vi "MainPanel.vi"() -> ()   [LabVIEW 2015]
uses:
  C:/Users/hskinner-bahay/Documents/GitHub/Kent_State_Project/Labview/LaserControl/SlugHFVInterface/SlugHFVInterface/bin/Debug/SlugHFVInterface.dll
  SlugHFVInterface/SlugHFVInterface/bin/Debug/SlugHFVInterface.dll
  <vilib>/Instr/_visa.llb/VISA Configure Serial Port (Instr).vi
panel:
  in  "Pulse Spacing":u8(knob) max=60 step=10 scale=0.0..60.0
  in  "Pulse Duration":u8(knob) max=60 step=10 scale=0.0..60.0
  in  "Duty Cycle":u8(knob)=100 max=100 step=50 scale=0.0..100.0
  in  "Power Level":u8(knob)=5 max=10 step=1 scale=0.0..10.0
  out "Power On Indicator":u32(colorbox)
  out "Fault LED":bool
  in  "Stop Button 3":bool
  in  "Start Button":bool
  in  "Stop Button":bool
  in  "Load Settings Button":bool
  in  "Saved Settings Field":string(combo)
  in  "Save Settings Button":bool
  in  "Save Settings Field":string
  out "Duty Cycle Slide":u8(slide) scale=0.0..100.0
  out "Slide 2":u8(slide) scale=0.0..100.0
  in  "Load Treatment Field":string(combo)
  in  "Instructions Dialog":bool
  out "Power Level Slide":u8(slide) max=100 step=5 scale=0.0..100.0
  in  "Tab Control":T1(tab)
  out "Strength Slide":u8(slide) scale=0.0..100.0
  out "Internlock LED":bool
  out "Temperature Slide":u8(slide) scale=0.0..100.0
  out "Power On LED":bool
  out "Cooling System LED":bool
  out "RF Active LED":bool
  in  "Numeric":dbl
  in  "Numeric 2":dbl
  in  "OK Button 7":bool
  in  "OK Button 8":bool
  in  "Numeric 3":dbl
  in  "Numeric 4":dbl
  out "Numeric 5":dbl
  out "Numeric 6":dbl
  out "Numeric 7":dbl
  out "Numeric 8":dbl
  in  "String 2":string
  in  "OK Button 5":bool
  in  "HFV Interface":refnum<visa-resource-name>
  # "HFV and Laser Control Panel"
  # "Pulse Duration"
  # "Power On"
  # "Stop"
  # "Power Level"
  # "Duty Cycle"
  # "Pulse Spacing"
  # "Begin Treatment"
  # "Load Treatment"
  # "Settings"
  # "Subject Temperature"
  # "Power On"
  # "Abort"
  # "Warning"
  # "Strength"
  # "Cooling System"
  # "Interlock"
  # "RF Active"
  # "Subject Temperature"
  # "Abort Cutoff (K)"
  # "Warning Cutoff (K)"
  # "Thermo Camera"
  # "Bounding Box"
  # "Measurement Filter (K)"
  # "High"
  # "Low"
  # "Thermo Camera"
  # "Save Readings"
  # "1"
  # "Probes"
  # "2"
  # "3"
  # "HFV Port (COM)"
  # "HFV Interface Circuit (COM)"
  # "Thermo Camera"
  # "Water Chiller Status (COM)"
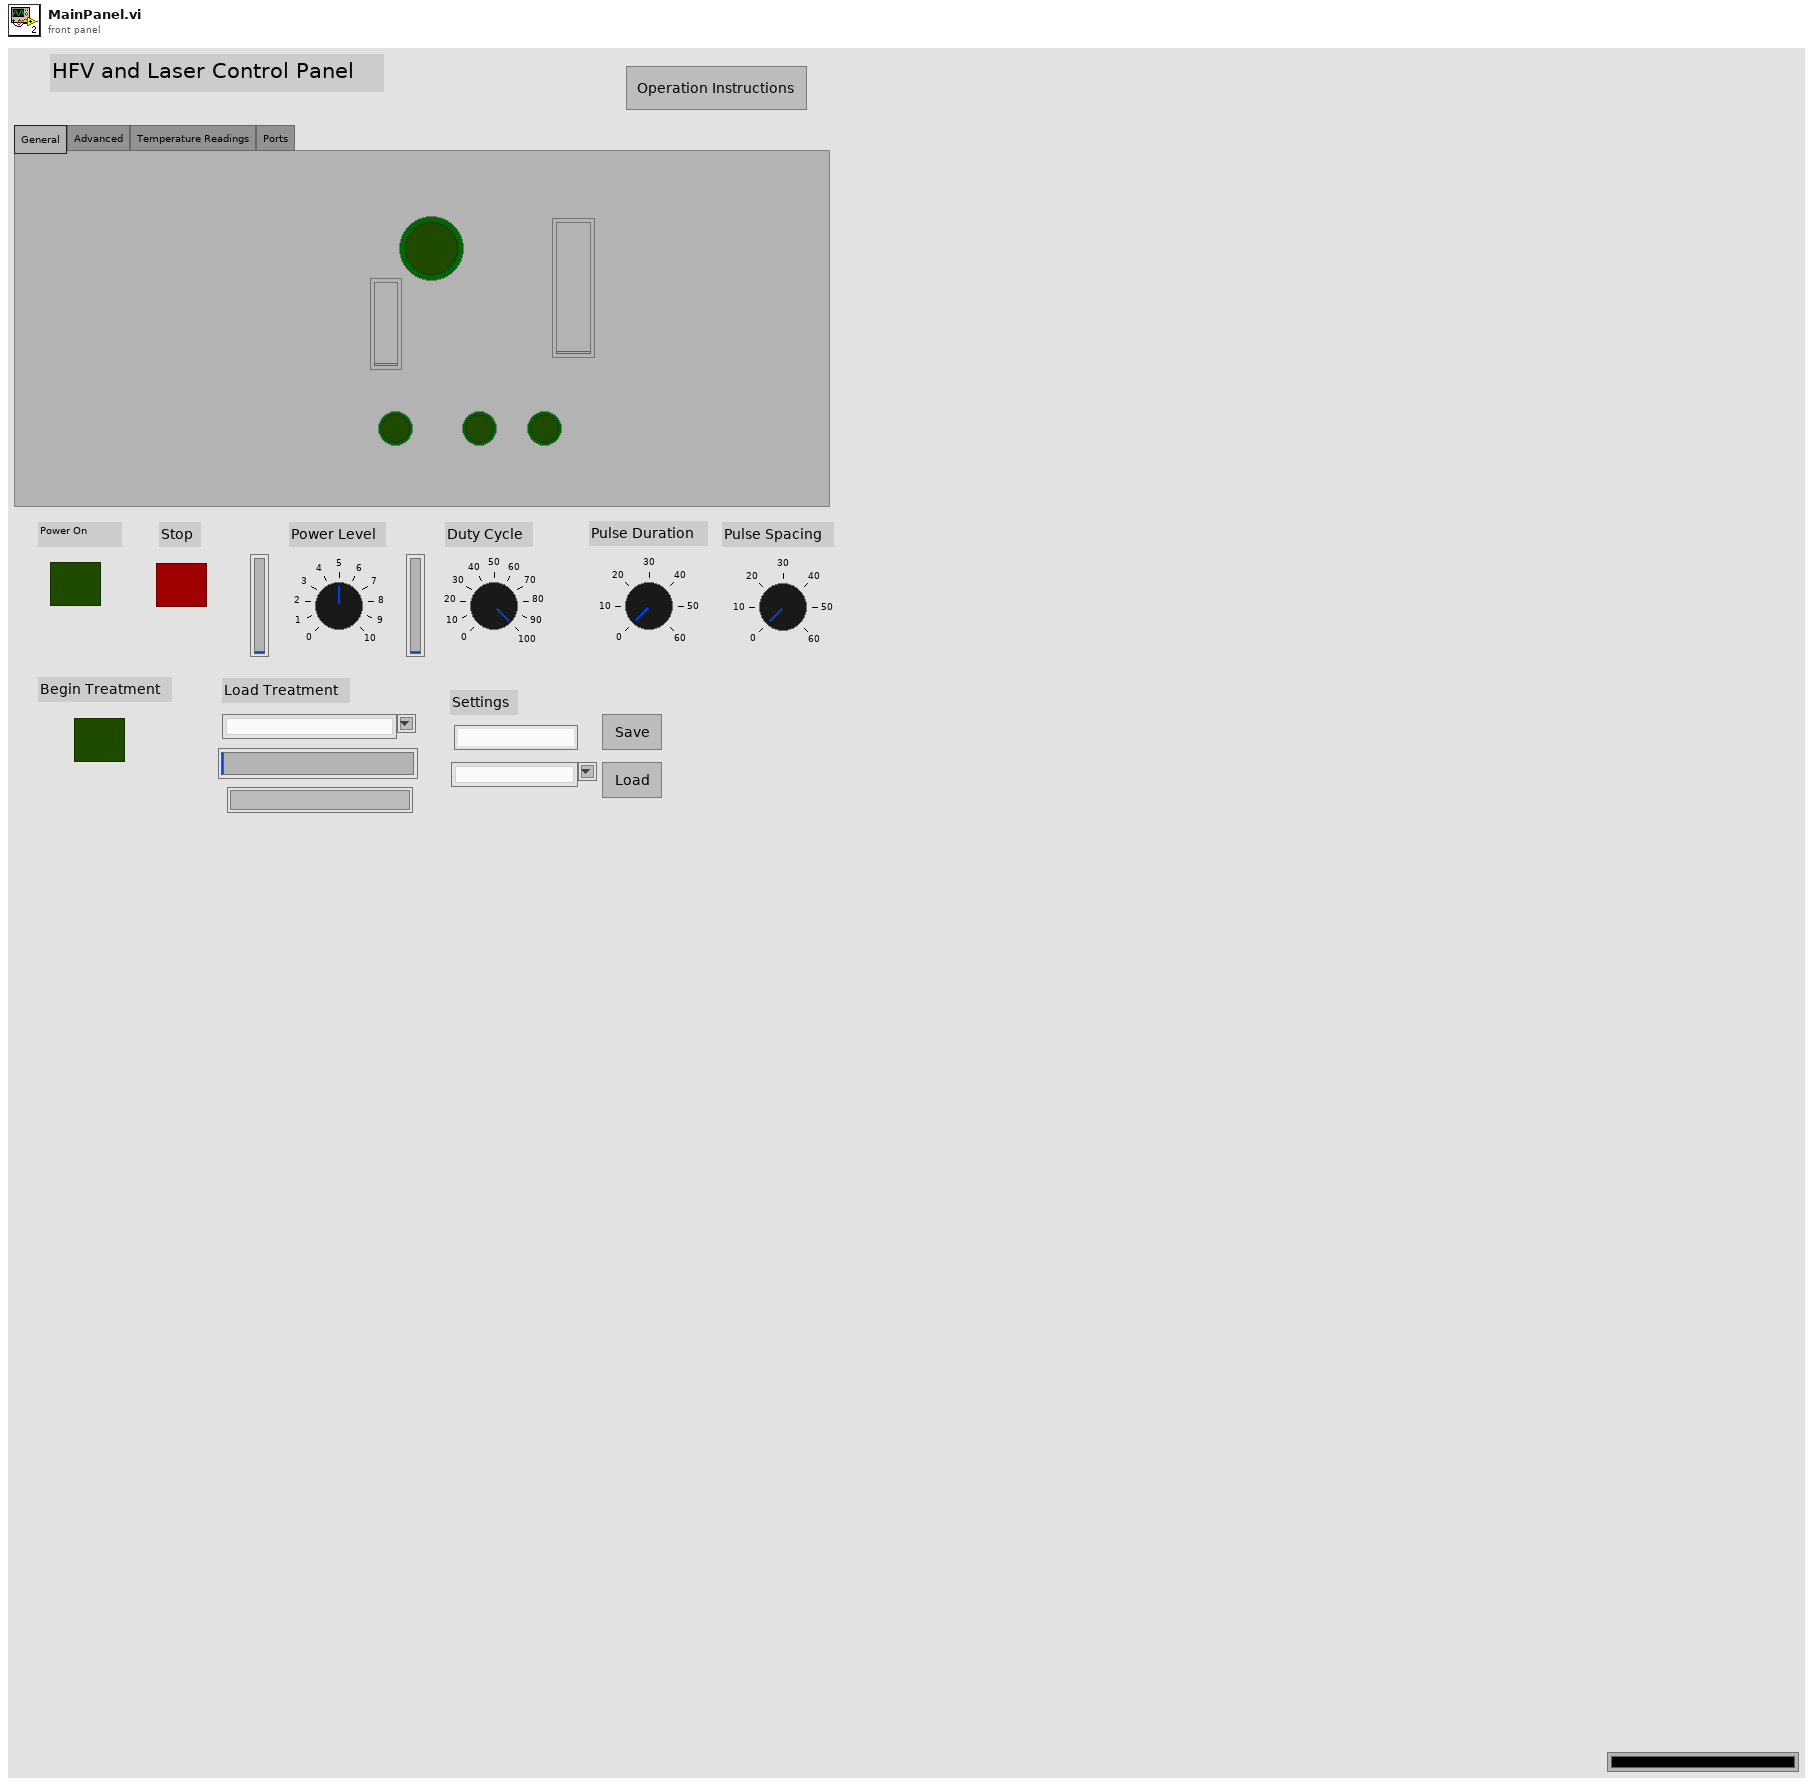
[diagram p1: front panel]
types:
  T1 = enum32{"General", "Advanced", "Temperature Readings", "Ports"}
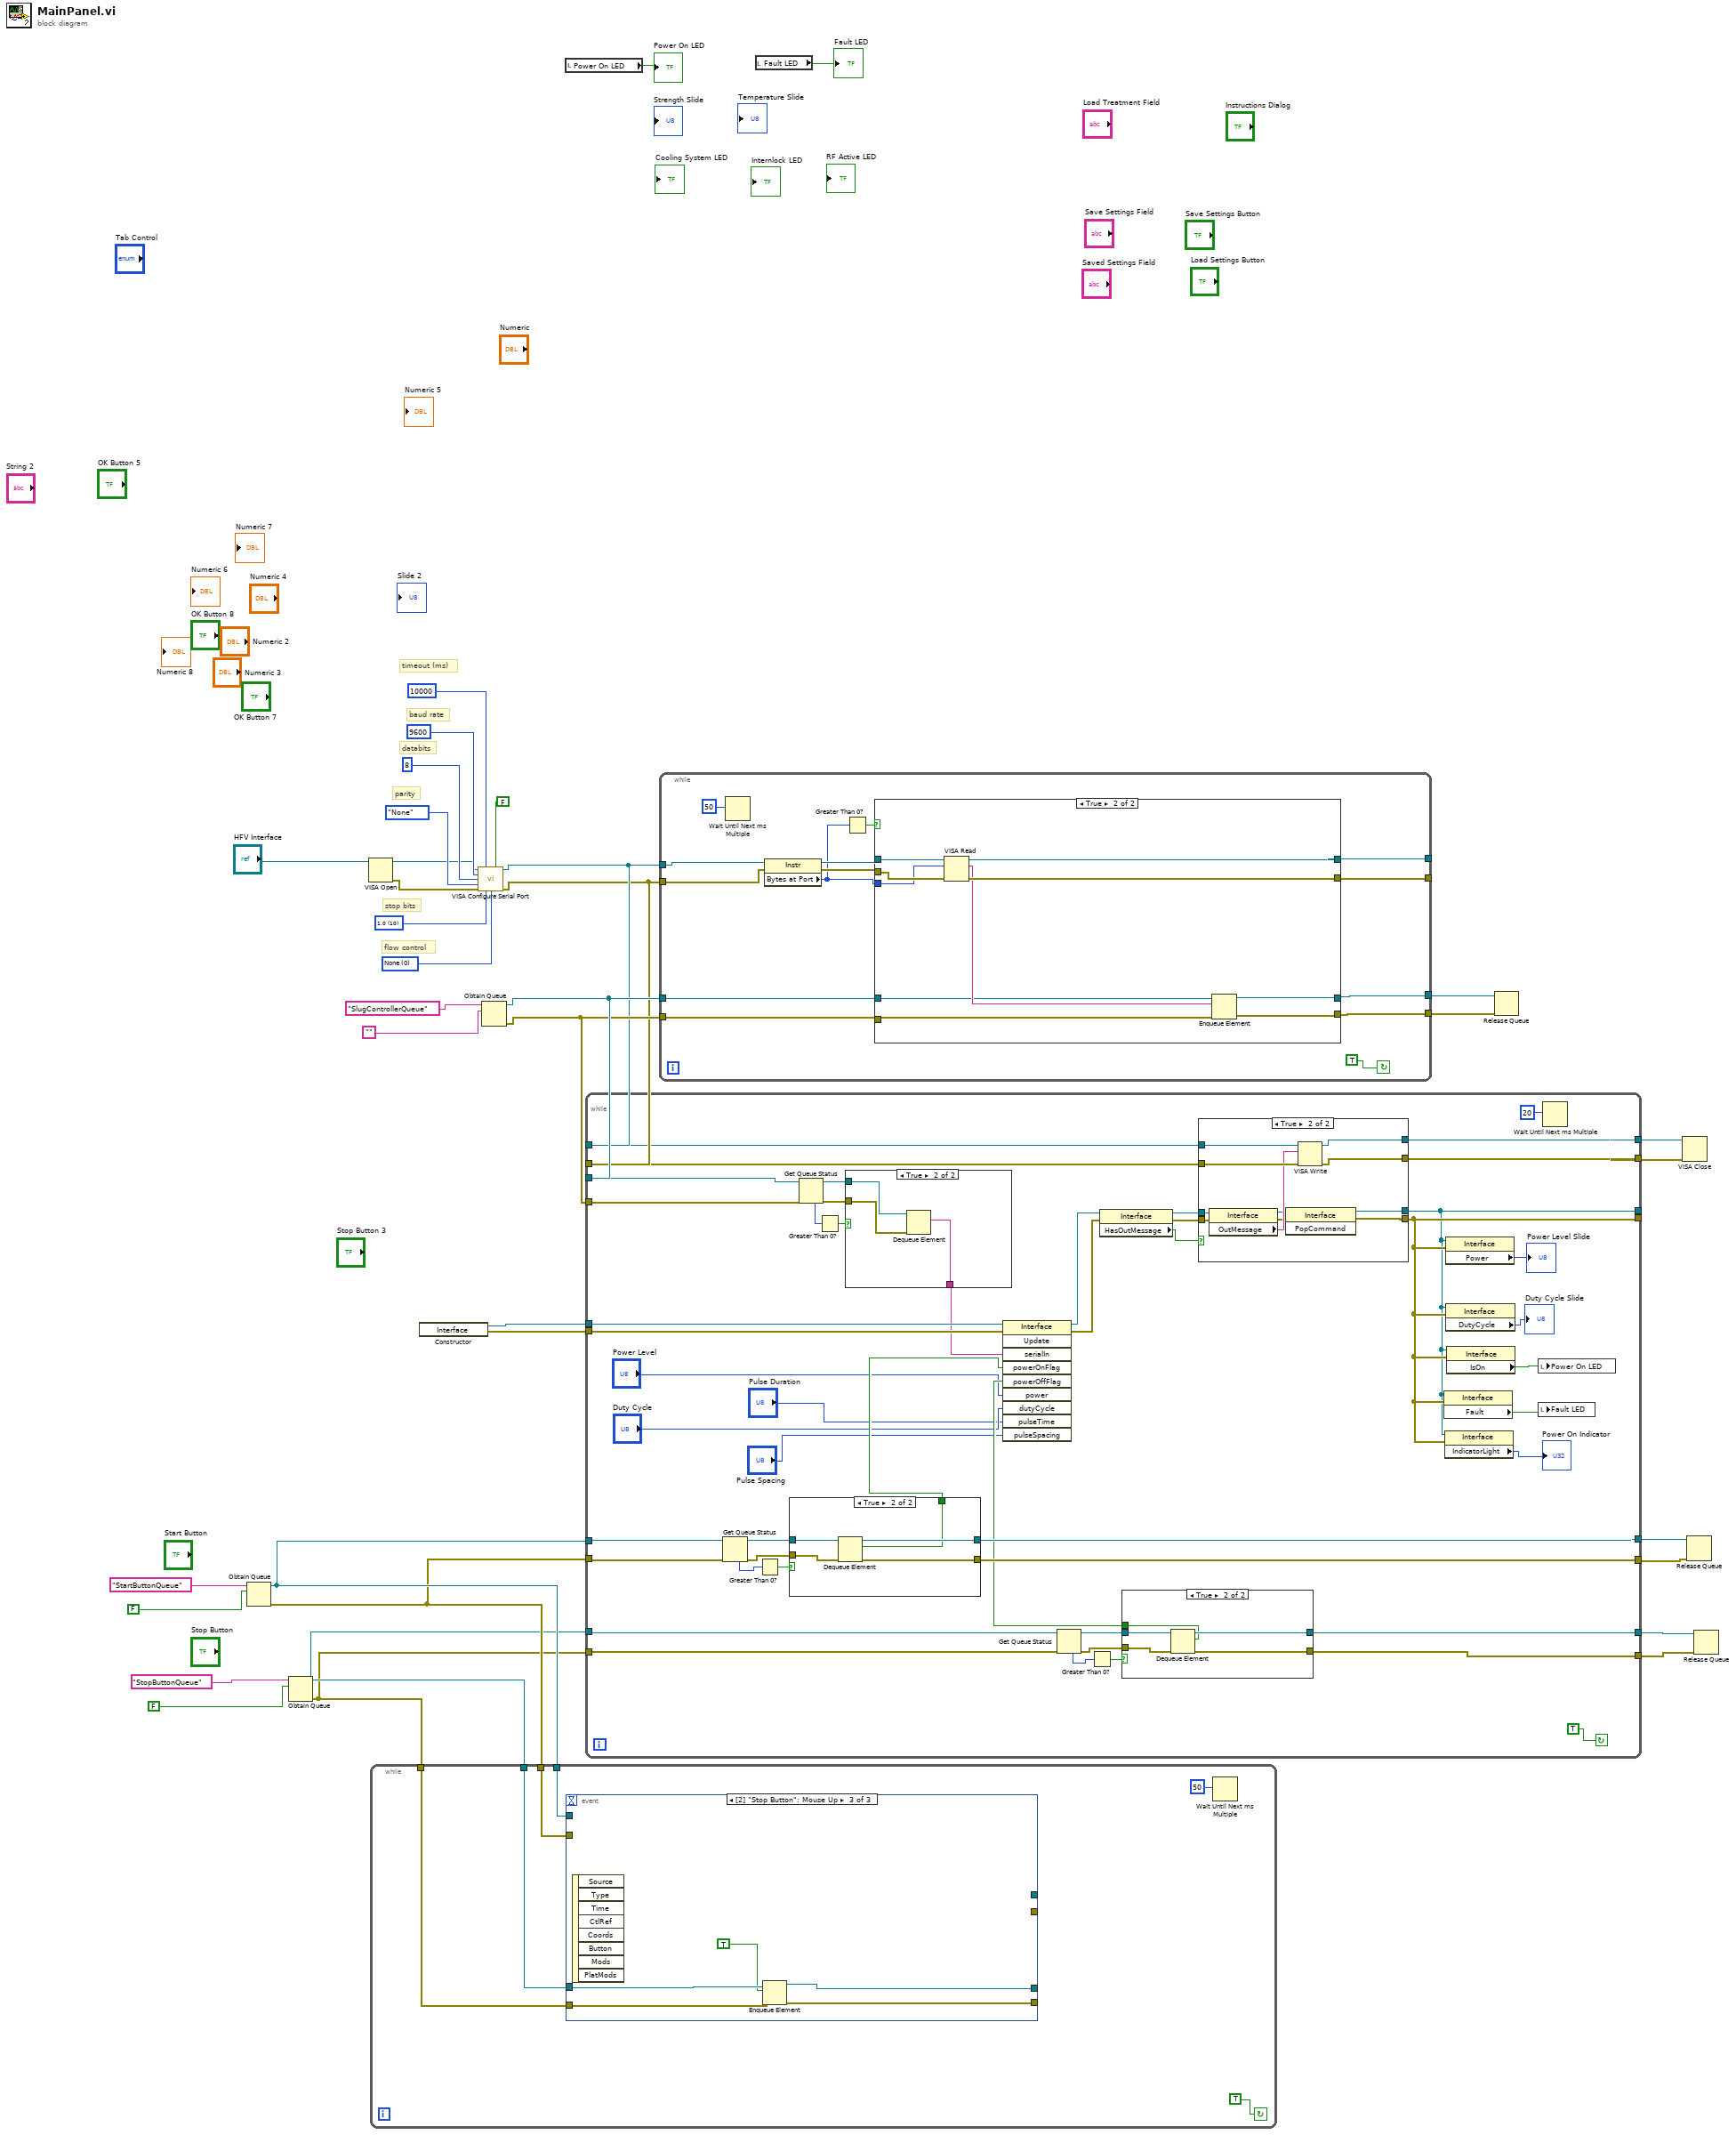
[diagram p0: block diagram]
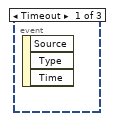
[diagram p2: hidden frame]
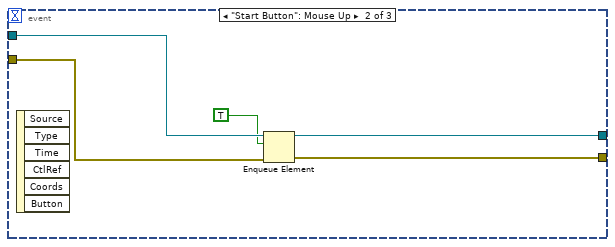
[diagram p3: hidden frame]
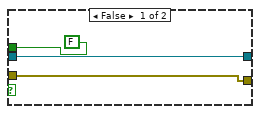
[diagram p4: hidden frame]
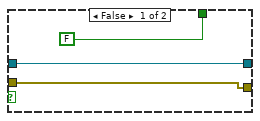
[diagram p5: hidden frame]
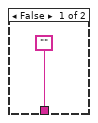
[diagram p7: hidden frame]
diagram:
  w32 = u16 0 items=["None", "XON/XOFF", "RTS/CTS", "XON/XOFF & RTS/CTS", "DTR/DSR", "XON/XOFF & DTR/DSR"] ("flow control (0:none)")
  w33 = u16 10 items=["1.0"=10, "1.5"=15, "2.0"=20] ("stop bits (10: 1 bit)")
  # "stop bits"
  # "flow control"
  # "parity"
  # "databits"
  # "baud rate"
  # "timeout (ms)"
  n1 = Obtain Queue(name (unnamed)="StartButtonQueue", element data type=FALSE) -> (queue out=w10:refnum<queue>, error out=w9:errorcluster)  [unwired: 3 in, 1 out]
  n2 = Obtain Queue(name (unnamed)="StopButtonQueue", element data type=FALSE) -> (queue out=w8:refnum<queue>, error out=w7:errorcluster)  [unwired: 3 in, 1 out]
  n3 = VISA Open(VISA resource name="HFV Interface") -> (VISA resource name=w29:refnum<visa-resource-name>, error out=w28:errorcluster)  [unwired: 4 in]
  n4 = while {
    tunnel: w10 -> [w42]
    tunnel: w9 -> [w41]
    tunnel: w8 -> [w40]
    tunnel: w7 -> [w39]
    stop <- TRUE continue-if-true
    n5 = event shown="[2] \"Stop Button\": Mouse Up" {
      selector: _ -> [_ _ _]
      dyn-events: _ -> [_ _ _]
      timeout: _ -> [_ _ _]
      tunnel: w42 -> [_ w47 _]
      tunnel: [_ w46 _] -> _
      tunnel: [_ w45 _] -> _
      tunnel: w41 -> [_ w44 _]
      tunnel: w40 -> [_ _ w52]
      tunnel: w39 -> [_ _ w51]
      tunnel: [_ _ w50] -> _
      tunnel: [_ _ w49] -> _
      event Timeout {
        n6 = event-data() -> ()  [unwired: 1 in, 3 out]
      }
      event "Start Button": Mouse Up {
        n7 = event-data() -> ()  [unwired: 1 in, 6 out]
        n8 = Enqueue Element(queue=w47, element=TRUE, error in (no error)=w44) -> (queue out=w46:refnum<queue>, error out=w45:errorcluster)  [unwired: 1 in, 1 out]
      }
      event "Stop Button": Mouse Up {
        n9 = event-data() -> ()  [unwired: 1 in, 8 out]
        n10 = Enqueue Element(queue=w52, element=TRUE, error in (no error)=w51) -> (queue out=w50:refnum<queue>, error out=w49:errorcluster)  [unwired: 1 in, 1 out]
      }
    }
    n11 = Wait Until Next ms Multiple(millisecond multiple=50) -> ()  [unwired: 1 out]
  }
  n12 = constructor class="Interface"() -> (reference out=w20:refnum<k24>, error out=w19:errorcluster)  [unwired: 3 in, 1 out]
  n13 = call-poly "VISA Configure Serial Port"("VISA resource name"=w29, "timeout (10sec)"=10000, "Enable Termination\nChar (T)"=FALSE ("Enable Termination\nChar (T)"), "baud rate (9600)"=9600, "data bits (8)"=8, "parity (0:none)"=enum16{"None", "Odd", "Even", "Mark", "Space"}."None", "error in (no error)"=w28, "stop bits (10: 1 bit)"=w33, "flow control (0:none)"=w32) -> ("VISA resource name out"=w18:refnum<visa-resource-name>, "error out"=w17:errorcluster)  [unwired: 5 in]
  n14 = Obtain Queue(name (unnamed)="SlugControllerQueue", element data type="") -> (queue out=w22:refnum<queue>, error out=w21:errorcluster)  [unwired: 3 in, 1 out]
  n15 = local read "Power On LED"() -> (→"Power On LED":bool)
  n16 = while {
    tunnel: w22 -> [w100]
    tunnel: w21 -> [w99]
    tunnel: w20 -> [w96]
    tunnel: w19 -> [w95]
    tunnel: w18 -> [w87]
    tunnel: w17 -> [w86]
    tunnel: [w60] -> _
    tunnel: [w61] -> _
    tunnel: [w83] -> w16
    tunnel: [w82] -> w15
    tunnel: w10 -> [w78]
    tunnel: w9 -> [w77]
    tunnel: [w74] -> w6
    tunnel: [w73] -> w5
    tunnel: w8 -> [w68]
    tunnel: w7 -> [w67]
    tunnel: [w66] -> w4
    tunnel: [w65] -> w3
    stop <- TRUE continue-if-true
    n17 = Get Queue Status(queue=w78, error in (no error)=w77) -> (queue out=w76:refnum<queue>, error out=w75:errorcluster, # elements in queue=w79:i32)  [unwired: 1 in, 5 out]
    n18 = Greater Than 0?(x=w79) -> (x > 0?=w80:bool)
    n19 = case shown="True" w80 {
      tunnel: w76 -> [w112 w117]
      tunnel: w75 -> [w111 w116]
      tunnel: [w112 w115] -> w74
      tunnel: [w111 w114] -> w73
      tunnel: [FALSE w113] -> w63
      frame False {
      }
      frame True {
        n20 = Dequeue Element(queue=w117, error in (no error)=w116) -> (queue out=w115:refnum<queue>, element=w113:bool, error out=w114:errorcluster)  [unwired: 1 in, 1 out]
      }
    }
    n21 = Get Queue Status(queue=w100, error in (no error)=w99) -> (queue out=w93:refnum<queue>, error out=w92:errorcluster, # elements in queue=w97:i32)  [unwired: 1 in, 5 out]
    n22 = Greater Than 0?(x=w97) -> (x > 0?=w98:bool)
    n23 = case shown="True" w98 {
      tunnel: ["" w134] -> w94
      tunnel: w93 -> [_ w136]
      tunnel: w92 -> [_ w135]
      frame False {
      }
      frame True {
        n24 = Dequeue Element(queue=w136, error in (no error)=w135) -> (element=w134:string)  [unwired: 1 in, 3 out]
      }
    }
    n25 = Get Queue Status(queue=w68, error in (no error)=w67) -> (queue out=w70:refnum<queue>, error out=w69:errorcluster, # elements in queue=w71:i32)  [unwired: 1 in, 5 out]
    n26 = Greater Than 0?(x=w71) -> (x > 0?=w72:bool)
    n27 = case shown="True" w72 {
      tunnel: w70 -> [w104 w109]
      tunnel: w69 -> [w103 w108]
      tunnel: [w104 w107] -> w66
      tunnel: [w103 w106] -> w65
      tunnel: [FALSE w105] -> w64
      frame False {
      }
      frame True {
        n28 = Dequeue Element(queue=w109, error in (no error)=w108) -> (queue out=w107:refnum<queue>, element=w105:bool, error out=w106:errorcluster)  [unwired: 1 in, 1 out]
      }
    }
    n29 = invoke class="Interface" method="Update"(reference=w96, error in=w95, "serialIn"=w94, "powerOnFlag"=w63, "powerOffFlag"=w64, "power"="Power Level", "dutyCycle"="Duty Cycle", "pulseTime"="Pulse Duration", "pulseSpacing"="Pulse Spacing") -> (reference out=w90:refnum<k24>, error out=w89:errorcluster)  [unwired: 1 in, 8 out]
    n30 = property class="Interface"(reference=w90, error in=w89) -> (reference out=w85:refnum<k24>, error out=w84:errorcluster, "HasOutMessage"=w88:bool)
    n31 = case shown="True" w88 {
      tunnel: w87 -> [w119 w132]
      tunnel: w86 -> [w118 w131]
      tunnel: w85 -> [w121 w130]
      tunnel: w84 -> [w120 w129]
      tunnel: [w121 w125] -> w60
      tunnel: [w120 w124] -> w61
      tunnel: [w119 w123] -> w83
      tunnel: [w118 w122] -> w82
      frame False {
      }
      frame True {
        n32 = property class="Interface"(reference=w130, error in=w129) -> (reference out=w127:refnum<k24>, error out=w126:errorcluster, "OutMessage"=w128:string)
        n33 = invoke class="Interface" method="PopCommand"(reference=w127, error in=w126) -> (reference out=w125:refnum<k24>, error out=w124:errorcluster)  [unwired: 1 in, 1 out]
        n34 = VISA Write(VISA resource name=w132, write buffer=w128, error in (no error)=w131) -> (VISA resource name out=w123:refnum<visa-resource-name>, error out=w122:errorcluster)  [unwired: 1 out]
      }
    }
    n35 = property class="Interface"(reference=w60, error in=w61) -> ("Fault"=w62:bool)  [unwired: 2 out]
    n36 = property class="Interface"(reference=w60, error in=w61) -> ("IndicatorLight"=→"Power On Indicator":i32)  [unwired: 2 out]
    n37 = property class="Interface"(reference=w60, error in=w61) -> ("Power"=→"Power Level Slide":i32)  [unwired: 2 out]
    n38 = property class="Interface"(reference=w60, error in=w61) -> ("DutyCycle"=→"Duty Cycle Slide":i32)  [unwired: 2 out]
    n39 = property class="Interface"(reference=w60, error in=w61) -> ("IsOn"=w81:bool)  [unwired: 2 out]
    n40 = local write "Power On LED"(w81) -> ()
    n41 = local write "Fault LED"(w62) -> ()
    n42 = Wait Until Next ms Multiple(millisecond multiple=20) -> ()  [unwired: 1 out]
  }
  n43 = while {
    tunnel: w18 -> [w139]
    tunnel: [w146] -> _
    tunnel: [w145] -> _
    tunnel: w22 -> [w137]
    tunnel: w21 -> [w142]
    tunnel: [w141] -> w26
    tunnel: [w140] -> w25
    tunnel: w17 -> [w138]
    stop <- TRUE continue-if-true
    n44 = Wait Until Next ms Multiple(millisecond multiple=50) -> ()  [unwired: 1 out]
    n45 = property class="Instr"(reference=w139, error in=w138) -> (reference out=w149:refnum<visa-resource-name>, error out=w150:errorcluster, "Bytes at Port"=w144:u32)
    n46 = Greater Than 0?(x=w144) -> (x > 0?=w148:bool)
    n47 = case shown="True" w148 {
      tunnel: w150 -> [w153 w164]
      tunnel: w149 -> [w154 w163]
      tunnel: [w154 w162] -> w146
      tunnel: [w153 w161] -> w145
      tunnel: w144 -> [_ w160]
      tunnel: w137 -> [w152 w158]
      tunnel: w142 -> [w151 w157]
      tunnel: [w152 w156] -> w141
      tunnel: [w151 w155] -> w140
      frame False {
      }
      frame True {
        n48 = VISA Read(VISA resource name=w163, byte count=w160, error in (no error)=w164) -> (VISA resource name out=w162:refnum<visa-resource-name>, read buffer=w159:string, error out=w161:errorcluster)  [unwired: 1 out]
        n49 = Enqueue Element(queue=w158, element=w159, error in (no error)=w157) -> (queue out=w156:refnum<queue>, error out=w155:errorcluster)  [unwired: 1 in, 1 out]
      }
    }
  }
  n50 = local read "Fault LED"() -> (→"Fault LED":bool)
  n51 = Release Queue(queue=w26, error in (no error)=w25) -> ()  [unwired: 1 in, 3 out]
  n52 = VISA Close(VISA resource name=w16, error in (no error)=w15) -> ()  [unwired: 1 out]
  n53 = Release Queue(queue=w6, error in (no error)=w5) -> ()  [unwired: 1 in, 3 out]
  n54 = Release Queue(queue=w4, error in (no error)=w3) -> ()  [unwired: 1 in, 3 out]
